vi "Write.vi"(1 "Connection":refnum<class "Connection.lvclass">, 3 "Close? (F)":bool, 4 "Element":T1, 5 "Timeout mS (-1)":i32) -> (0 "Closed?":bool, 2 "Timed Out?":bool)   [LabVIEW 2020, in "Connection.lvclass"]
uses:
  Connection.lvclass
  Element.ctl
  Connection.lvclass/Connection.ctl
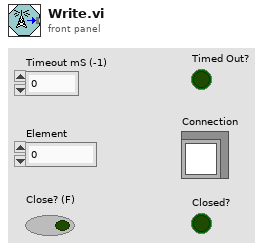
[diagram p1: front panel]
types:
  T1 = typedef "Connection.lvclass/Element.ctl" = dbl
  T2 = typedef "Connection.lvclass/Tag Data.ctl" = cluster{"Value":T1, "Updated":timestamp, "Sequence":u32}
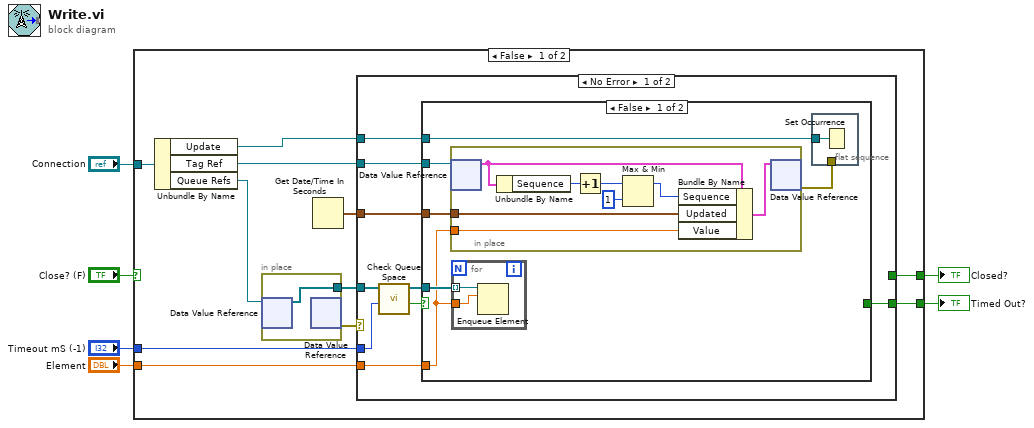
[diagram p0: block diagram]
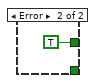
[diagram p3: hidden frame]
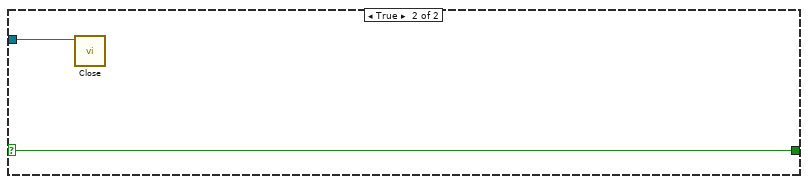
[diagram p4: hidden frame]
diagram:
  n1 = case shown="False" "Close? (F)" {
    selector: "Close? (F)" -> [_ w47]
    tunnel: "Connection" -> [w17 w48]
    tunnel: [w7 w47] -> w4
    tunnel: "Timeout mS (-1)" -> [w10 _]
    tunnel: "Element" -> [w8 _]
    tunnel: [w9 _] -> w1
    frame False {
      n2 = Unbundle By Name(w17) -> ("Update"=w12:refnum<k4>, "Tag Ref"=w13:refnum<data-value>, "Queue Refs"=w16:refnum<data-value>)
      n3 = in-place {
        in-place-border: [w46] -> w14
        n4 = in-place-dvr #1(w16) -> (w46:refnum<queue>[])  [unwired: 1 out]
        n5 = in-place-dvr #1() -> (w15:errorcluster)  [unwired: 1 in, 1 out]
      }
      n6 = Get Date/Time In Seconds() -> (seconds since 1Jan1904=w11:timestamp)
      n7 = case shown="No Error" w15 {
        tunnel: w14 -> [w26 _]
        tunnel: w13 -> [w20 _]
        tunnel: w12 -> [w19 _]
        tunnel: w11 -> [w22 _]
        tunnel: w10 -> [w25 _]
        tunnel: [w23 _] -> w9
        tunnel: w8 -> [w21 _]
        tunnel: [_ TRUE] -> w7
        frame No Error {
          n8 = call "Check Queue Space.vi"("Timeout mS"=w25, "Queues In"=w26) -> ("Timeout"=w24:bool, "Queues"=w18:refnum<queue>[])  [unwired: 8 in]
          n9 = case shown="False" w24 {
            selector: w24 -> [_ w44]
            tunnel: [_ w44] -> w23
            tunnel: w22 -> [w31 _]
            tunnel: w21 -> [w27 _]
            tunnel: w20 -> [w32 _]
            tunnel: w19 -> [w30 _]
            tunnel: w18 -> [w28 _]
            frame False {
              n10 = in-place {
                in-place-border: w31 -> [w38]
                in-place-border: w27 -> [w37]
                n11 = in-place-dvr #2(w32) -> (w40:T2)  [unwired: 1 out]
                n12 = Unbundle By Name(w40) -> ("Sequence"=w43:u32)
                n13 = Increment(x=w43) -> (x+1=w42:u32)
                n14 = Max & Min(x=w42, y=u32 1) -> (max(x,y)=w39:u32)  [unwired: 1 out]
                n15 = Bundle By Name(cluster=w40, "Sequence"=w39, "Updated"=w38, "Value"=w37) -> (w36:T2)
                n16 = in-place-dvr #2(w36) -> (w29:errorcluster)  [unwired: 1 out]
              }
              n17 = for {
                tunnel: w28 -> [w34] mode=indexing
                tunnel: w27 -> [w33]
                n18 = Enqueue Element(queue=w34, element=w33) -> ()  [unwired: 2 in, 3 out]
              }
              n19 = flat-sequence {
                tunnel: w30 -> [w35]
                tunnel: w29 -> [_]
                frame #0 {
                  n20 = Set Occurrence(w35) -> ()
                }
              }
            }
            frame True {
            }
          }
        }
        frame Error {
        }
      }
    }
    frame True {
      n21 = call "Close.vi"("Connection in"=w48) -> ()  [unwired: 9 in, 2 out]
    }
  }
  "Timed Out?" <- w1
  "Closed?" <- w4
